vi "Str_to_Ch_dis_ADAM.vi"(4 "String Row":string) -> (0 "Value":dbl format="%.2f", 1 "Ch Description":T1={"Ch Name"="", "Type"="", "Function"=enum."Analogue Input", "Ch State"=enum."On", "Calibration type"=enum."Raw", "A"=0.0, "B"=0.0, "C"=0.0, "D"=0.0, "Comments"="", "Address"={"Main"=0, "Ch."=0, "Sub"=0, "Port Name"=""}, "String"="", "Duty"=65535} {"Duty" format="%.0b"; "D" format="%#_5g"; "C" format="%#_5g"; "B" format="%#_5g"; "A" format="%#_5g"})   [LabVIEW 2012]
uses:
  ADAM Controls/Ch_description_ADAM.ctl
  ADAM Controls/Module_type_ADAM.ctl
  ADAM Controls/Function_ADAM.ctl
  ADAM Controls/Channel_State.ctl
  ADAM Controls/Calib_type_ADAM.ctl
  ADAM Controls/Address.ctl
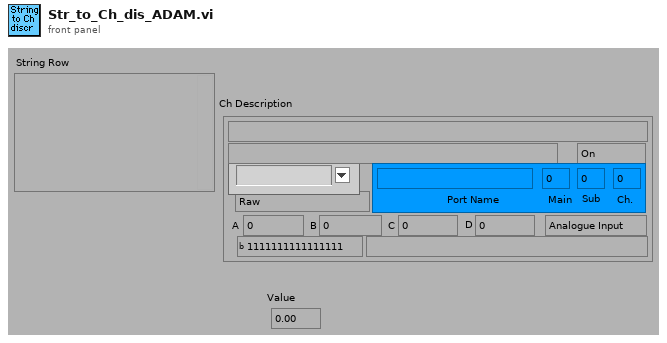
[diagram p1: front panel]
types:
  T1 = typedef "Ch_description_ADAM.ctl" = cluster{"Ch Name":string, "Type":T2, "Function":T3, "Ch State":T4, "Calibration type":T5, "A":dbl, "B":dbl, "C":dbl, "D":dbl, "Comments":string, "Address":T6, "String":string, "Duty":u16}
  T2 = typedef "Module_type_ADAM.ctl" = string
  T3 = typedef "Function_ADAM.ctl" = enum16{"Analogue Input", "Digital Input", "Event counter", "Event rate", "Analogue Output", "Digital Output", "Relay Output"}
  T4 = typedef "Channel_State.ctl" = enum16{"On", "Off", "Always On", "Always Off"}
  T5 = typedef "Calib_type_ADAM.ctl" = enum16{"Raw", "Bx + A", "Cx^2 + Bx + A", "Dx^3 + Cx^2 + Bx + A", "In Band", "Hi-Tec Q", "Hi-Tec M_dot", "Text"}
  T6 = typedef "Address.ctl" = cluster{"Main":i32, "Ch.":i32, "Sub":i32, "Port Name":string}
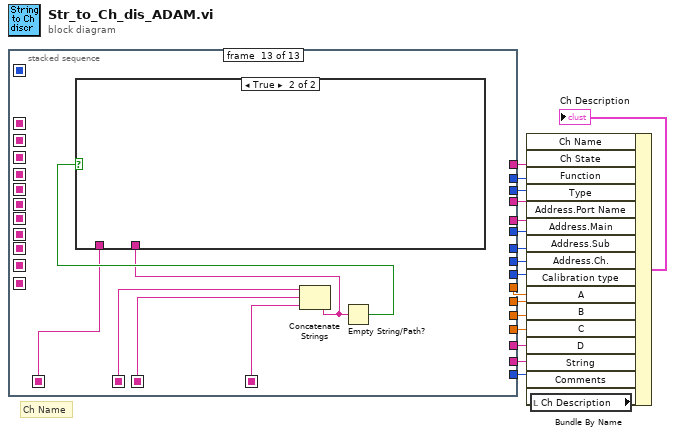
[diagram p0: block diagram]
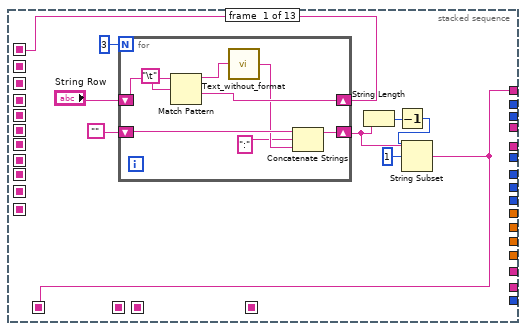
[diagram p2: hidden frame]
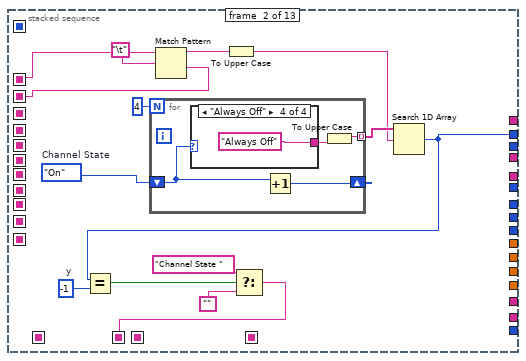
[diagram p3: hidden frame]
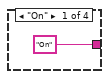
[diagram p4: hidden frame]
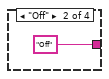
[diagram p5: hidden frame]
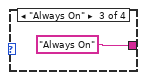
[diagram p6: hidden frame]
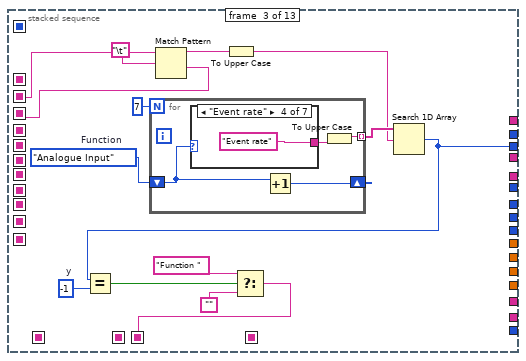
[diagram p7: hidden frame]
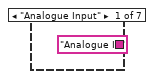
[diagram p8: hidden frame]
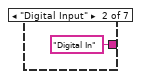
[diagram p9: hidden frame]
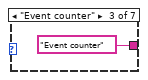
[diagram p10: hidden frame]
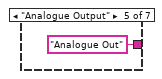
[diagram p11: hidden frame]
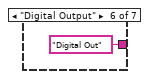
[diagram p12: hidden frame]
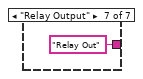
[diagram p13: hidden frame]
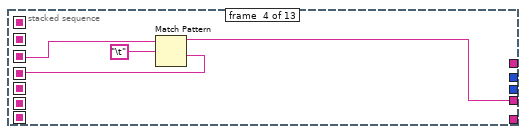
[diagram p14: hidden frame]
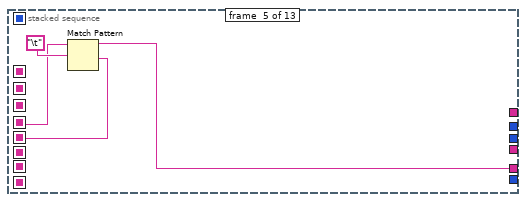
[diagram p15: hidden frame]
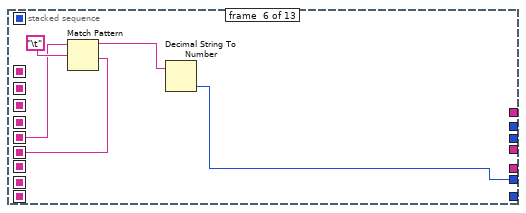
[diagram p16: hidden frame]
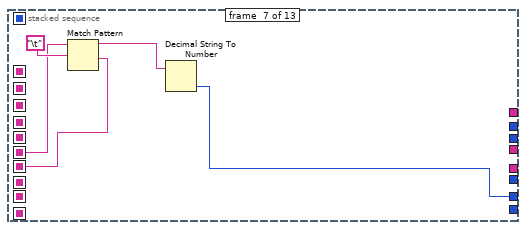
[diagram p17: hidden frame]
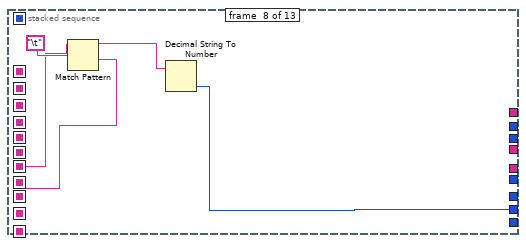
[diagram p18: hidden frame]
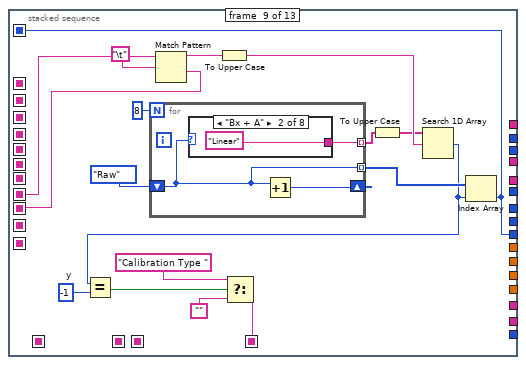
[diagram p19: hidden frame]
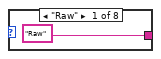
[diagram p20: hidden frame]
diagram:
  # "Ch Name"
  n1 = stacked-sequence {
    seq-local: [w24 _ _ _ _ _ _ _ _ _ _ _ _] -> [_ w43 _ _ _ _ _ _ _ _ _ _ _]
    seq-local: [_ w42 _ _ _ _ _ _ _ _ _ _ _] -> [_ _ w67 _ _ _ _ _ _ _ _ _ _]
    seq-local: [w19 _ _ _ _ _ _ _ _ _ _ _ _] -> [_ _ _ _ _ _ _ _ _ _ _ _ w167]
    seq-local: [_ _ w65 _ _ _ _ _ _ _ _ _ _] -> [_ _ _ w84 _ _ _ _ _ _ _ _ _]
    seq-local: [_ _ _ _ w89 _ _ _ _ _ _ _ _] -> [_ _ _ _ _ w93 _ _ _ _ _ _ _]
    seq-local: [_ _ _ _ _ _ _ w102 _ _ _ _ _] -> [_ _ _ _ _ _ _ _ w115 _ _ _ _]
    seq-local: [_ _ _ w85 _ _ _ _ _ _ _ _ _] -> [_ _ _ _ w88 _ _ _ _ _ _ _ _]
    seq-local: [_ _ _ _ _ _ _ _ _ w135 _ _ _] -> [_ _ _ _ _ _ _ _ _ _ w153 _ _]
    seq-local: [_ _ _ _ _ w92 _ _ _ _ _ _ _] -> [_ _ _ _ _ _ w98 _ _ _ _ _ _]
    seq-local: [_ _ _ _ _ _ w97 _ _ _ _ _ _] -> [_ _ _ _ _ _ _ w103 _ _ _ _ _]
    seq-local: [_ _ _ _ _ _ _ _ w114 _ _ _ _] -> [_ _ _ _ _ _ _ _ _ w134 _ _ _]
    seq-local: [_ _ _ _ _ _ _ _ _ _ w150 _ _] -> [_ _ _ _ _ _ _ _ _ _ _ w164 _]
    seq-local: [_ _ _ _ _ _ _ _ w110 _ _ _ _] -> [_ _ _ _ _ _ _ _ _ _ _ _ _]
    seq-local: [_ w36 _ _ _ _ _ _ _ _ _ _ _] -> [_ _ _ _ _ _ _ _ _ _ _ _ w171]
    seq-local: [_ _ w58 _ _ _ _ _ _ _ _ _ _] -> [_ _ _ _ _ _ _ _ _ _ _ _ w170]
    seq-local: [_ _ _ _ _ _ _ _ w106 _ _ _ _] -> [_ _ _ _ _ _ _ _ _ _ _ _ w166]
    tunnel: [_ _ w64 _ _ _ _ _ _ _ _ _ _] -> w18
    tunnel: [_ w40 _ _ _ _ _ _ _ _ _ _ _] -> w17
    tunnel: [_ _ _ _ w87 _ _ _ _ _ _ _ _] -> w14
    tunnel: [_ _ _ _ _ _ _ w101 _ _ _ _ _] -> w7
    tunnel: [_ _ _ _ _ _ _ _ w110 _ _ _ _] -> w8
    tunnel: [_ _ _ _ _ _ _ _ _ w147 _ _ _] -> w9
    tunnel: [_ _ _ _ _ _ _ _ _ w146 _ _ _] -> w10
    tunnel: [_ _ _ _ _ _ _ _ _ w145 _ _ _] -> w11
    tunnel: [_ _ _ _ _ _ _ _ _ w144 _ _ _] -> w12
    tunnel: [_ _ _ _ _ _ _ _ _ _ w154 _ _] -> w13
    tunnel: [w19 _ _ _ _ _ _ _ _ _ _ _ _] -> w15
    tunnel: [_ _ _ _ _ w91 _ _ _ _ _ _ _] -> w6
    tunnel: [_ _ _ _ _ _ w96 _ _ _ _ _ _] -> w5
    tunnel: [_ _ _ _ _ _ _ _ _ _ w148 _ _] -> w3
    tunnel: [_ _ _ _ _ _ _ _ _ _ _ w159 _] -> w2
    tunnel: [_ _ _ w83 _ _ _ _ _ _ _ _ _] -> w1
    frame #0 {
      n2 = for {
        N: 3 -> [_]
        shift-right: [w33] -> w24
        shift-left: "String Row" -> [w34]
        shift-right: [w30] -> w23
        shift-left: "" -> [w31]
        n3 = Match Pattern(string=w34, regular expression="\t") -> (before substring=w32:string, after substring=w33:string)  [unwired: 3 out]
        n4 = call "Text_without_format.vi"("Input string"=w32) -> ("Output string"=w29:string)
        n5 = Concatenate Strings(w31, ":" ("String without format char"), w29) -> (w30:string)
      }
      n6 = String Length(string=w23) -> (length=w22:i32)
      n7 = Decrement(x=w22) -> (x-1=w21:i32)
      n8 = String Subset(string=w23, offset (0)=1, length (rest)=w21) -> (substring=w19:string)
    }
    frame #1 {
      w41 = Channel_State."On"  # Channel State
      w46 = -1  # y
      n9 = for {
        N: 4 -> [_]
        shift-right: [w53] -> _
        shift-left: w41 -> [w51]
        tunnel: [w52] -> w48 mode=indexing
        n10 = case shown="\"Always Off\"" w51 {
          tunnel: ["On" "Off" "Always On" "Always Off"] -> w50
          frame "On" {
          }
          frame "Off" {
          }
          frame "Always On" {
          }
          frame "Always Off" {
          }
        }
        n11 = Increment(x=w51) -> (x+1=w53:T4)
        n12 = To Upper Case(1:w50) -> (0:w52:string)
      }
      n13 = Match Pattern(string=w43, regular expression="\t") -> (before substring=w45:string, after substring=w42:string)  [unwired: 3 out]
      n14 = To Upper Case(1:w45) -> (0:w44:string)
      n15 = Search 1D Array(1D array=w48, element=w44) -> (index of element=w40:i32)  [unwired: 1 out]
      n16 = Equal?(x=w40, y=w46) -> (x = y?=w37:bool)
      n17 = Select(t="Channel State ", s=w37, f="") -> (s? t:f=w36:string)
    }
    frame #2 {
      w62 = Function_ADAM."Analogue Input"  # Function
      w68 = -1  # y
      n18 = for {
        N: 7 -> [_]
        shift-right: [w75] -> _
        shift-left: w62 -> [w73]
        tunnel: [w74] -> w70 mode=indexing
        n19 = case shown="\"Event rate\"" w73 {
          tunnel: ["Analogue In" "Digital In" "Event counter" "Event rate" "Analogue Out" "Digital Out" "Relay Out"] -> w72
          frame "Analogue Input" {
          }
          frame "Digital Input" {
          }
          frame "Event counter" {
          }
          frame "Event rate" {
          }
          frame "Analogue Output" {
          }
          frame "Digital Output" {
          }
          frame "Relay Output" {
          }
        }
        n20 = Increment(x=w73) -> (x+1=w75:T3)
        n21 = To Upper Case(1:w72) -> (0:w74:string)
      }
      n22 = Match Pattern(string=w67, regular expression="\t") -> (before substring=w66:string, after substring=w65:string)  [unwired: 3 out]
      n23 = To Upper Case(1:w66) -> (0:w63:string)
      n24 = Search 1D Array(1D array=w70, element=w63) -> (index of element=w64:i32)  [unwired: 1 out]
      n25 = Equal?(x=w64, y=w68) -> (x = y?=w59:bool)
      n26 = Select(t="Function ", s=w59, f="") -> (s? t:f=w58:string)
    }
    frame #3 {
      n27 = Match Pattern(string=w84, regular expression="\t") -> (before substring=w83:string, after substring=w85:string)  [unwired: 3 out]
    }
    frame #4 {
      n28 = Match Pattern(string=w88, regular expression="\t") -> (before substring=w87:string, after substring=w89:string)  [unwired: 3 out]
    }
    frame #5 {
      n29 = Match Pattern(string=w93, regular expression="\t") -> (before substring=w94:string, after substring=w92:string)  [unwired: 3 out]
      n30 = Decimal String To Number(string=w94) -> (number=w91:i32)  [unwired: 3 out]
    }
    frame #6 {
      n31 = Match Pattern(string=w98, regular expression="\t") -> (before substring=w99:string, after substring=w97:string)  [unwired: 3 out]
      n32 = Decimal String To Number(string=w99) -> (number=w96:i32)  [unwired: 3 out]
    }
    frame #7 {
      n33 = Match Pattern(string=w103, regular expression="\t") -> (before substring=w104:string, after substring=w102:string)  [unwired: 3 out]
      n34 = Decimal String To Number(string=w104) -> (number=w101:i32)  [unwired: 3 out]
    }
    frame #8 {
      w119 = -1  # y
      n35 = for {
        N: 8 -> [_]
        shift-right: [w125] -> _
        shift-left: Calib_type_ADAM."Raw" ("Calibration Type") -> [w123]
        tunnel: [w124] -> w121 mode=indexing
        tunnel: [w123] -> w112 mode=indexing
        n36 = case shown="\"Bx + A\"" w123 {
          tunnel: ["Raw" "Linear" "Quad" "Cubic" "In Band" "Hi-Tec Q" "Hi-Tec M_dot" "Text"] -> w124
          frame "Raw" {
          }
          frame "Bx + A" {
          }
          frame "Cx^2 + Bx + A" {
          }
          frame "Dx^3 + Cx^2 + Bx + A" {
          }
          frame "In Band" {
          }
          frame "Hi-Tec Q" {
          }
          frame "Hi-Tec M_dot" {
          }
          frame "Text" {
          }
        }
        n37 = Increment(x=w123) -> (x+1=w125:T5)
      }
      n38 = Match Pattern(string=w115, regular expression="\t") -> (before substring=w118:string, after substring=w114:string)  [unwired: 3 out]
      n39 = To Upper Case(1:w118) -> (0:w117:string)
      n40 = To Upper Case(1:w121) -> (0:w116:string[])
      n41 = Search 1D Array(1D array=w116, element=w117) -> (index of element=w111:i32)  [unwired: 1 out]
      n42 = Equal?(x=w111, y=w119) -> (x = y?=w107:bool)
      n43 = Select(t="Calibration Type ", s=w107, f="") -> (s? t:f=w106:string)
      n44 = Index Array(array=w112, index=w111) -> (element=w110:T5)
    }
    frame #9 {
      w142 = "\t"
      n45 = Match Pattern(string=w134, regular expression=w142) -> (before substring=w139:string, after substring=w143:string)  [unwired: 3 out]
      n46 = Match Pattern(string=w143, regular expression=w142) -> (before substring=w138:string, after substring=w141:string)  [unwired: 3 out]
      n47 = Match Pattern(string=w141, regular expression=w142) -> (before substring=w137:string, after substring=w140:string)  [unwired: 3 out]
      n48 = Match Pattern(string=w140, regular expression=w142) -> (before substring=w136:string, after substring=w135:string)  [unwired: 3 out]
      n49 = Fract/Exp String To Number(string=w138) -> (number=w146:dbl)  [unwired: 4 out]
      n50 = Fract/Exp String To Number(string=w137) -> (number=w145:dbl)  [unwired: 4 out]
      n51 = Fract/Exp String To Number(string=w139) -> (number=w147:dbl)  [unwired: 4 out]
      n52 = Fract/Exp String To Number(string=w136) -> (number=w144:dbl)  [unwired: 4 out]
    }
    frame #10 {
      n53 = Match Pattern(string=w153, regular expression="\t") -> (before substring=w155:string, after substring=w151:string)  [unwired: 3 out]
      n54 = Match Pattern(string=w151, regular expression="\t") -> (before substring=w149:string, after substring=w150:string)  [unwired: 3 out]
      n55 = call "Text_without_format.vi"("Input string"=w155) -> ("Output string"=w154:string)
      n56 = call "Text_without_format.vi"("Input string"=w149) -> ("Output string"=w148:string)
    }
    frame #11 {
      n57 = Match Pattern(string=w164, regular expression="\t") -> (before substring=w157:string, after substring=w161:string)  [unwired: 3 out]
      n58 = Match Pattern(string=w161, regular expression="\t") -> (before substring=w158:string)  [unwired: 4 out]
      n59 = Fract/Exp String To Number(string=w158) -> (number=→"Value":dbl)  [unwired: 4 out]
      n60 = Decimal String To Number(string=w157) -> (number=w160:i32)  [unwired: 3 out]
      n61 = To Unsigned Word Integer(number=w160) -> (unsigned 16bit integer=w159:u16)
    }
    frame #12 {
      n62 = Concatenate Strings(w171, w170, w166) -> (w168:string)
      n63 = Empty String/Path?(string/path=w168) -> (empty?=w169:bool)
      n64 = case shown="True" w169 {
        tunnel: w168 -> [w178 _]
        tunnel: w167 -> [w176 _]
        frame False {
          w172 = TRUE  # Dialog Box
          n65 = Concatenate Strings(w178, "Invalid for ch named ", w176) -> (w175:string)
          n66 = Bundle By Name(cluster=errorcluster {"status"=FALSE, "code"=0, "source"=""} ("error in (no error)"), "status"=TRUE ("Bundle Element"), "source"=w175) -> (w173:errorcluster)
          n67 = call "EnFlo_Error_Handler.vi"("error in (no error)"=w173, "Dialog Box (T)"=w172) -> ()  [unwired: 1 in, 3 out]
        }
        frame True {
        }
      }
    }
  }
  n68 = local read "Ch Description"() -> (w16:T1)
  n69 = Bundle By Name(cluster=w16, "Ch Name"=w15, "Ch State"=w17, "Function"=w18, "Type"=w1, "Address.Port Name"=w14, "Address.Main"=w6, "Address.Sub"=w5, "Address.Ch."=w7, "Calibration type"=w8, "A"=w9, "B"=w10, "C"=w11, "D"=w12, "String"=w13, "Comments"=w3, "Duty"=w2) -> (→"Ch Description":T1)
